vi "15.2.1 GeoWithCalibriation.vi"() -> ()   [LabVIEW 2016]
uses:
  <vilib>/vision/Image Controls.llb/IMAQ Image.ctl
  <vilib>/vision/Pattern Matching.llb/IMAQ GM Match Report.ctl
  <vilib>/vision/Pattern Matching.llb/IMAQ Match Range Setting.ctl
  <vilib>/vision/NI_Vision_Development_Module.lvlib
panel:
  out "Calibration":T1(plugin-control)
  out "#of Matches":i32
  out "UUT":T1(plugin-control)
  out "Feature":T1(plugin-control)
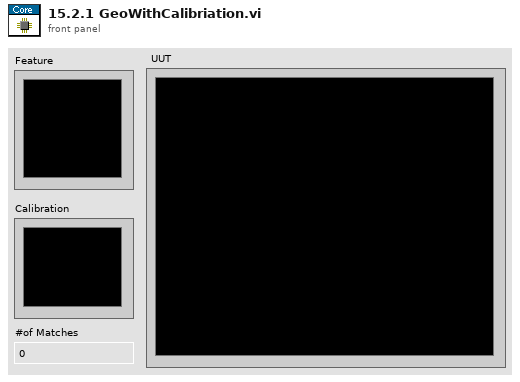
[diagram p1: front panel]
types:
  T1 = typedef "IMAQ Image.ctl" = refnum<image>
  T2 = cluster{"Setup Data Item":u16, "Item Value":dbl}[]
  T3 = typedef "IMAQ Match Range Setting.ctl" = cluster{"Match Constraints":u32, "Min":dbl, "Max":dbl}
  T4 = cluster{"Rotation":bool, "Scale":bool, "Occlusion":bool, "Reserved":bool, "Reserved":bool, "Reserved":bool}
  T5 = typedef "IMAQ GM Match Report.ctl" = cluster{"Position":cluster{"x":sgl, "y":sgl}, "Angle":sgl, "Scale":sgl, "Score":sgl, "Bounding Box":cluster{"x":sgl, "y":sgl}[], "Contrast Reversed":bool, "Occlusion %":sgl, "Template Target Curve Score":sgl, "Target Template Curve Score":sgl, "Correlation Score":sgl}
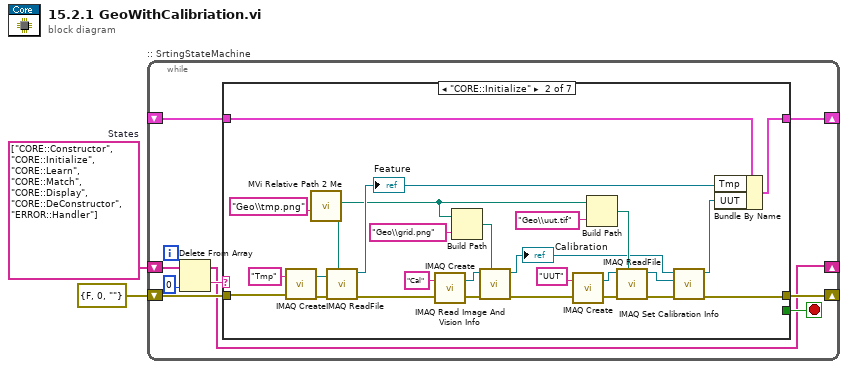
[diagram p0: block diagram]
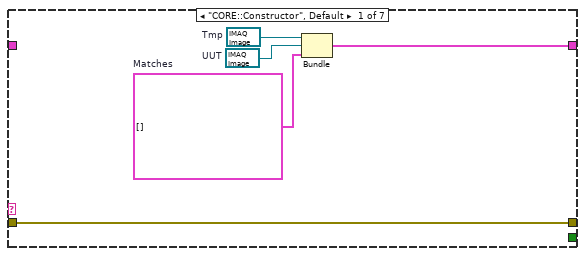
[diagram p2: hidden frame]
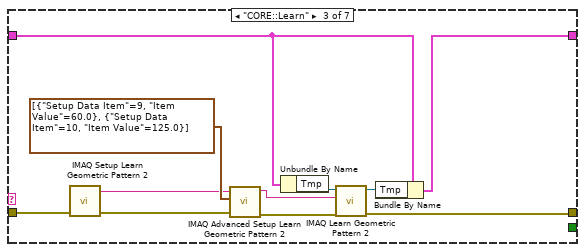
[diagram p3: hidden frame]
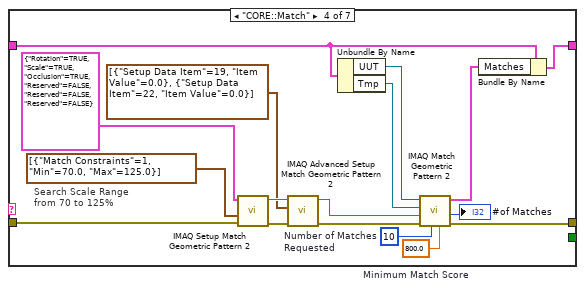
[diagram p4: hidden frame]
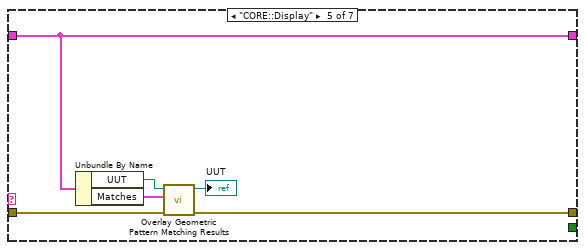
[diagram p5: hidden frame]
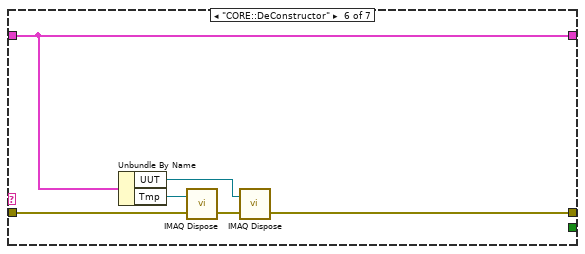
[diagram p6: hidden frame]
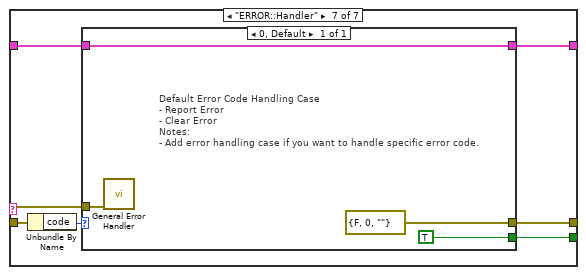
[diagram p7: hidden frame]
diagram:
  w1 = string[] ["CORE::Constructor", "CORE::Initialize", "CORE::Learn", "CORE::Match", "CORE::Display", "CORE::DeConstructor", "ERROR::Handler"]  # States
  n1 = while ":: SrtingStateMachine" {
    shift-right: [w8] -> _
    shift-left: errorcluster {"status"=FALSE, "code"=0, "source"=""} ("ErrI") -> [w6]
    shift-right: [w10] -> _
    shift-left: _ -> [w9]
    shift-right: [w3] -> _
    shift-left: w1 -> [w7]
    stop <- w11 stop-if-true
    n2 = Delete From Array(array=w7, index=0) -> (deleted portion=w5:string, array with subset deleted=w3:string[])  [unwired: 1 in]
    n3 = case shown="\"CORE::Initialize\"" w5 {
      tunnel: [w15 w25 w47 w64 w76 w79 w86] -> w8
      tunnel: [_ _ _ _ _ _ w85] -> w11
      tunnel: w6 -> [w15 w38 w48 w69 w77 w83 w84]
      tunnel: [w16 w41 w53 w59 w74 w82 w87] -> w10
      tunnel: w9 -> [_ w42 w54 w60 w74 w82 w88]
      frame "CORE::Constructor", Default {
        w12 = T5[] []  # Matches
        w13 = T1 refnum  # UUT
        w14 = T1 refnum  # Tmp
        n4 = Bundle("Tmp"=w14, "UUT"=w13, "Matches"=w12) -> (w16:cluster{"Tmp":T1, "UUT":T1, "Matches":T5[]})  [unwired: 1 in]
      }
      frame "CORE::Initialize" {
        n5 = call "IMAQ Create"("Image Name"="Tmp", "error in (no error)"=w38) -> ("Src"=w40:T1, "error out"=w39:errorcluster)  [unwired: 3 in]
        n6 = call "MVi Relative Path 2 Me.vi"("Relative Path"="Geo\\tmp.png" ("name or relative path")) -> ("Appended Dir"=w33:path, "MyDir"=w20:path)  [unwired: 5 in]
        n7 = call "IMAQ ReadFile"("File Path"=w33, "error in (no error)"=w39, "Image"=w40) -> ("error out"=w28:errorcluster, "Image Out"=w32:T1)  [unwired: 4 in, 3 out]
        "Feature" <- w32
        n8 = call "IMAQ Create"("Image Name"="Cal", "error in (no error)"=w28) -> ("Src"=w29:T1, "error out"=w30:errorcluster)  [unwired: 3 in]
        n9 = Build Path(base path=w20, name or relative path="Geo\\grid.png") -> (appended path=w22:path)
        n10 = call "IMAQ Read Image And Vision Info"("File Path"=w22, "error in (no error)"=w30, "Image"=w29) -> ("error out"=w27:errorcluster, "Image Out"=w17:T1)  [unwired: 6 in, 1 out]
        "Calibration" <- w17
        n11 = call "IMAQ Create"("Image Name"="UUT", "error in (no error)"=w27) -> ("Src"=w35:T1, "error out"=w36:errorcluster)  [unwired: 3 in]
        n12 = Build Path(base path=w20, name or relative path="Geo\\uut.tif") -> (appended path=w19:path)
        n13 = call "IMAQ ReadFile"("File Path"=w19, "error in (no error)"=w36, "Image"=w35) -> ("error out"=w26:errorcluster, "Image Out"=w24:T1)  [unwired: 4 in, 3 out]
        n14 = call "IMAQ Set Calibration Info"("error in (no error)"=w26, "Image Dst"=w24, "Image Src"=w17) -> ("error out"=w25:errorcluster, "Calibrated Image"=w18:T1)  [unwired: 7 in]
        n15 = Bundle By Name(cluster=w42, "Tmp"=w32, "UUT"=w18) -> (w41:cluster{"Tmp":T1, "UUT":T1, "Matches":T5[]})
      }
      frame "CORE::Learn" {
        n16 = call "IMAQ Setup Learn Geometric Pattern 2"("error in (no error)"=w48) -> ("error out"=w50:errorcluster, "Learn Geometric Pattern 2 Setup Data"=w49:string)  [unwired: 1 in]
        n17 = call "IMAQ Advanced Setup Learn Geometric Pattern 2"("Learn Geometric Pattern 2 Setup Data In"=w49, "Advanced Geometric Learn Options 2"=T2 [{"Setup Data Item"=9, "Item Value"=60.0}, {"Setup Data Item"=10, "Item Value"=125.0}], "error in (no error)"=w50) -> ("Learn Geometric Pattern 2 Setup Data Out"=w46:string, "error out"=w51:errorcluster)  [unwired: 6 in]
        n18 = Unbundle By Name(w54) -> ("Tmp"=w45:T1)
        n19 = call "IMAQ Learn Geometric Pattern 2"("error in (no error)"=w51, "Learn Geometric Pattern 2 Setup Data"=w46, "Template Image"=w45) -> ("error out"=w47:errorcluster, "Template Image Out"=w44:T1)  [unwired: 7 in]
        n20 = Bundle By Name(cluster=w54, "Tmp"=w44) -> (w53:cluster{"Tmp":T1, "UUT":T1, "Matches":T5[]})
      }
      frame "CORE::Match" {
        w56 = sgl 800.0  # Minimum Match Score
        w57 = 10  # Number of Matches Requested
        # "Search Scale Range from 70 to 125%"
        n21 = call "IMAQ Setup Match Geometric Pattern 2"("error in (no error)"=w69, "Range Settings"=T3[] [{"Match Constraints"=1, "Min"=70.0, "Max"=125.0}], "Match Mode"=T4 {"Rotation"=TRUE, "Scale"=TRUE, "Occlusion"=TRUE, "Reserved"=FALSE, "Reserved"=FALSE, "Reserved"=FALSE}) -> ("error out"=w66:errorcluster, "Match Geometric Pattern 2 Setup Data"=w68:string)  [unwired: 7 in]
        n22 = call "IMAQ Advanced Setup Match Geometric Pattern 2"("Match Geometric Pattern 2 Setup Data In"=w68, "Advanced Geometric Match Options 2"=T2 [{"Setup Data Item"=19, "Item Value"=0.0}, {"Setup Data Item"=22, "Item Value"=0.0}], "error in (no error)"=w66) -> ("Match Geometric Pattern 2 Setup Data Out"=w63:string, "error out"=w65:errorcluster)  [unwired: 6 in]
        n23 = Unbundle By Name(w60) -> ("UUT"=w62:T1, "Tmp"=w61:T1)
        n24 = call "IMAQ Match Geometric Pattern 2"("Minimum Match Score"=w56, "Number of Matches Requested"=w57, "error in (no error)"=w65, "Match Geometric Pattern 2 Setup Data"=w63, "Template Image"=w61, "Image"=w62) -> ("error out"=w64:errorcluster, "Number of Matches"=→"#of Matches":i32, "Matches (pixel)"=w58:T5[])  [unwired: 1 in, 2 out]
        n25 = Bundle By Name(cluster=w60, "Matches"=w58) -> (w59:cluster{"Tmp":T1, "UUT":T1, "Matches":T5[]})
      }
      frame "CORE::Display" {
        n26 = Unbundle By Name(w74) -> ("UUT"=w73:T1, "Matches"=w72:T5[])
        n27 = call "Overlay Geometric Pattern Matching Results.vi"("error in"=w77, "Matches"=w72, "Image"=w73) -> ("error out"=w76:errorcluster, "Image Out"=→"UUT":T1)  [unwired: 2 in, 5 out]
      }
      frame "CORE::DeConstructor" {
        n28 = Unbundle By Name(w82) -> ("UUT"=w78:T1, "Tmp"=w81:T1)
        n29 = call "IMAQ Dispose"("Image"=w81, "error in (no error)"=w83) -> ("error out"=w80:errorcluster)  [unwired: 4 in]
        n30 = call "IMAQ Dispose"("Image"=w78, "error in (no error)"=w80) -> ("error out"=w79:errorcluster)  [unwired: 4 in]
      }
      frame "ERROR::Handler" {
        n31 = Unbundle By Name(w84) -> ("code"=w89:i32)
        n32 = case shown="0, Default" w89 {
          tunnel: [w93] -> w87
          tunnel: w88 -> [w93]
          tunnel: [errorcluster {"status"=FALSE, "code"=0, "source"=""} ("error out")] -> w86
          tunnel: [TRUE] -> w85
          tunnel: w84 -> [w91]
          frame 0, Default {
            # "Default Error Code Handling Case\n- Report Error\n- Clear Error \nNotes:\n- Add error handling case if you want to handle specific error code."
            n33 = call <vilib>:"General Error Handler.vi"("error in (no error)"=w91) -> ()  [unwired: 10 in, 5 out]
          }
        }
      }
    }
  }
